vi "writeObject.vi"(8 "error in (no error)":errorcluster, 9 "rf.lvclass":refnum<class "rf.lvclass">, 10 "Array":refnum<class "rf.lvclass">[](array[class]), 11 "rfArray in":refnum<class "rfArray.lvclass">) -> (0 "error out":errorcluster, 2 "Array out":refnum<class "rf.lvclass">[](array[class]), 3 "rfArray out":refnum<class "rfArray.lvclass">)   [LabVIEW 2009, in "Tools.lvlib" / "Scripting.lvlib" / "rfArray.lvclass"]
uses:
  rfArray.lvclass
  Rf Event/rf.lvclass
  DatabaseHelpers/Database Objects/Channel/Channel.lvclass
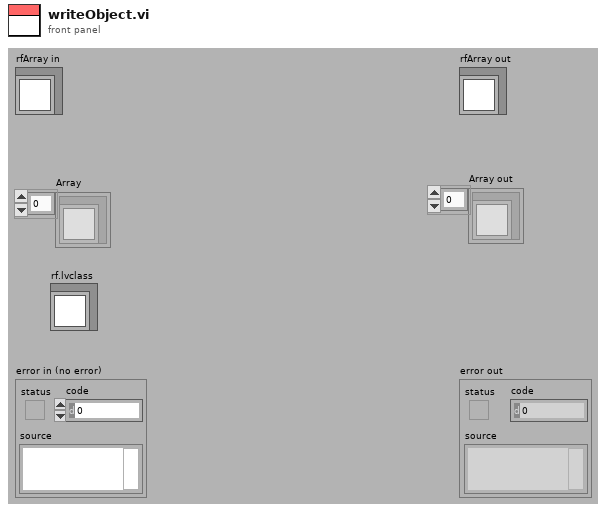
[diagram p1: front panel]
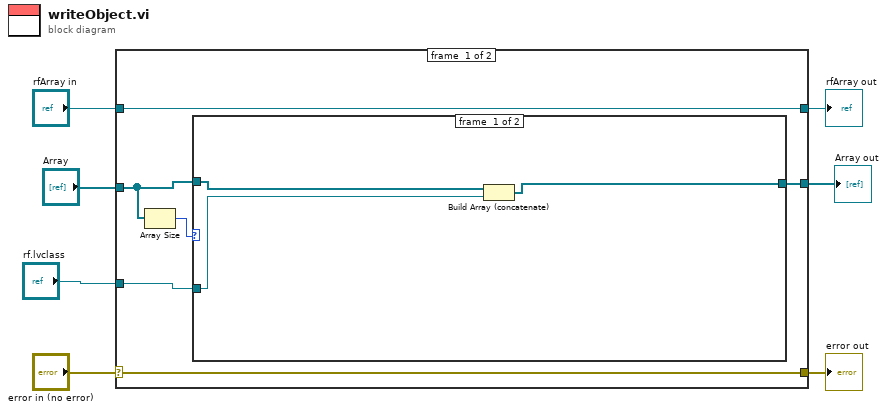
[diagram p0: block diagram]
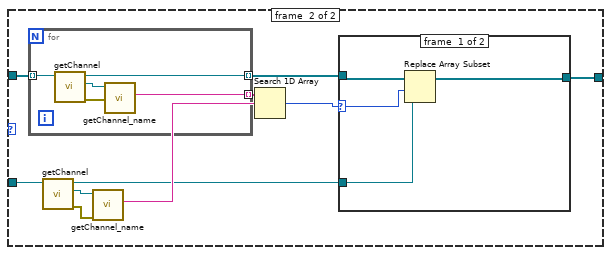
[diagram p2: hidden frame]
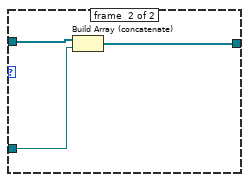
[diagram p3: hidden frame]
diagram:
  n1 = case shown="No Error" "error in (no error)" {
    selector: "error in (no error)" -> [w12 w40]
    tunnel: [w12 w40] -> w6
    tunnel: [w13 w39] -> w4
    tunnel: "rfArray in" -> [w13 w39]
    tunnel: "Array" -> [w9 _]
    tunnel: "rf.lvclass" -> [w11 _]
    tunnel: [w10 _] -> w1
    frame #0 {
      n2 = Array Size(array=w9) -> (size(s)=w8:i32)
      n3 = case shown="Default" w8 {
        tunnel: w11 -> [w15 w25]
        tunnel: [w14 w18] -> w10
        tunnel: w9 -> [w16 w17]
        frame #0 {
          n4 = Build Array (concatenate)(w16, w15) -> (w14:refnum<class "rf.lvclass">[])
        }
        frame #1 {
          n5 = for {
            tunnel: w17 -> [w36] mode=indexing
            tunnel: [w35] -> w23 mode=indexing
            tunnel: [w34] -> w20 mode=indexing
            n6 = call-dynamic "getChannel.vi"("ScriptEvent.lvclass in"=w36) -> ("error out"=w37:errorcluster, "Channel.lvclass"=w38:refnum<class "Channel.lvclass">, "ScriptEvent.lvclass out"=w34:refnum<class "rf.lvclass">)  [unwired: 8 in]
            n7 = call "getChannel_name.vi"("error in (no error)"=w37, "Channel.lvclass in"=w38) -> ("channel_name"=w35:string)  [unwired: 7 in, 2 out]
          }
          n8 = call-dynamic "getChannel.vi"("ScriptEvent.lvclass in"=w25) -> ("error out"=w24:errorcluster, "Channel.lvclass"=w26:refnum<class "Channel.lvclass">, "ScriptEvent.lvclass out"=w19:refnum<class "rf.lvclass">)  [unwired: 8 in]
          n9 = call "getChannel_name.vi"("error in (no error)"=w24, "Channel.lvclass in"=w26) -> ("channel_name"=w22:string)  [unwired: 7 in, 2 out]
          n10 = Search 1D Array(1D array=w23, element=w22) -> (index of element=w21:i32)  [unwired: 1 in]
          n11 = case shown="0, Default" w21 {
            selector: w21 -> [w29 _]
            tunnel: w20 -> [w30 w33]
            tunnel: w19 -> [w28 w32]
            tunnel: [w27 w31] -> w18
            frame #0 {
              n12 = Replace Array Subset(array=w30, new element=w28, index=w29) -> (w27:refnum<class "rf.lvclass">[])
            }
            frame #1 {
              n13 = Build Array (concatenate)(w33, w32) -> (w31:refnum<class "rf.lvclass">[])
            }
          }
        }
      }
    }
    frame #1 {
    }
  }
  "error out" <- w6
  "rfArray out" <- w4
  "Array out" <- w1
